vi "Wait for Completion.vi"(8 "error in (no error)":errorcluster, 9 "Timeout":i32, 11 "Coverage Analyzer Process in":refnum<class "Coverage Analyzer Process.lvclass">) -> (0 "error out":errorcluster, 3 "Coverage Analyzer Process out":refnum<class "Coverage Analyzer Process.lvclass">)   [LabVIEW 2020, in "Coverage Analyzer Process.lvclass"]
uses:
  Coverage Analyzer Process.lvclass
  Coverage Analyzer Process.lvclass/Coverage Analyzer Process.ctl
  Coverage Analyzer Result View/Coverage Analyzer View Data.ctl
  Coverage Analyzer Result View/Coverage Analyzer View.vi
  Coverage Analyzer Result View/Coverage Analyzer Result View.lvclass
  Coverage Analyzer/Coverage Analyzer.lvclass
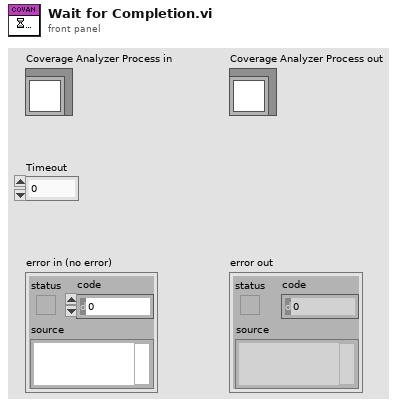
[diagram p1: front panel]
types:
  T1 = typedef "Coverage Analyzer Result View.lvclass/Coverage Analyzer View Data.ctl" = cluster{"Code Coverage":map{path, dbl}}
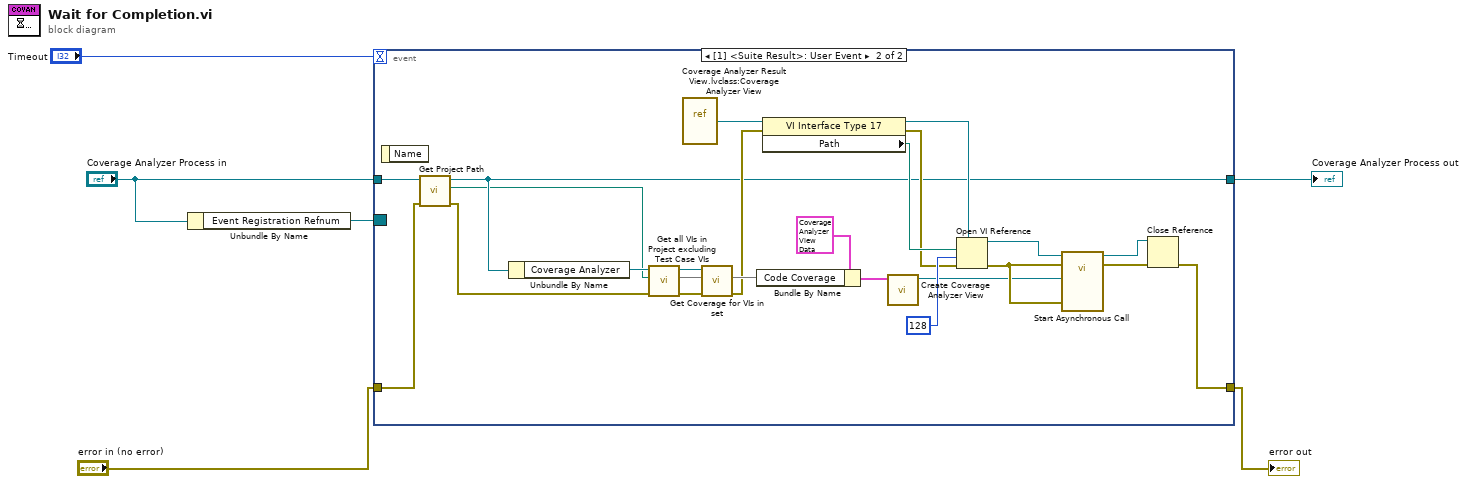
[diagram p0: block diagram]
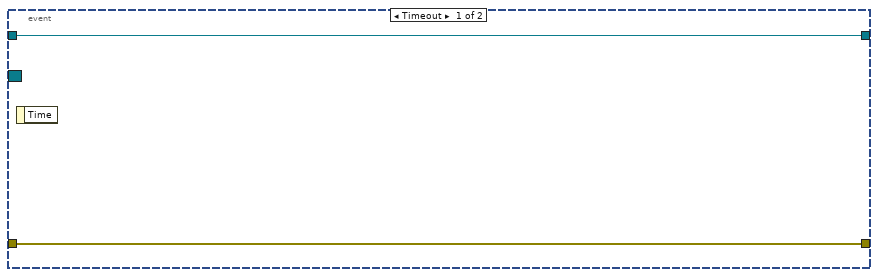
[diagram p2: hidden frame]
diagram:
  n1 = Unbundle By Name("Coverage Analyzer Process in") -> ("Event Registration Refnum"=w5:refnum<event-registration>)
  n2 = event shown="[1] <Suite Result>: User Event" {
    selector: w5 -> [_ _]
    dyn-events: _ -> [_ _]
    timeout: "Timeout" -> [_ _]
    tunnel: "error in (no error)" -> [w8 w13]
    tunnel: [w8 w23] -> w3
    tunnel: "Coverage Analyzer Process in" -> [w7 w15]
    tunnel: [w7 w16] -> w1
    event Timeout {
      n3 = event-data() -> ()  [unwired: 1 in, 1 out]
    }
    event User Event {
      n4 = event-data() -> ()  [unwired: 1 in, 1 out]
      n5 = call "Get Project Path.vi"("error in (no error)"=w13, "Coverage Analyzer Process in"=w15) -> ("error out"=w14:errorcluster, "Path"=w10:path, "Coverage Analyzer Process out"=w16:refnum<class "Coverage Analyzer Process.lvclass">)  [unwired: 7 in]
      n6 = Unbundle By Name(w16) -> ("Coverage Analyzer"=w21:refnum<class "Coverage Analyzer.lvclass">)
      n7 = call "Get all VIs in Project excluding Test Case VIs.vi"("error in (no error)"=w14, "Path"=w10, "Coverage Analyzer in"=w21) -> ("error out"=w18:errorcluster, "VIs"=w9:set{path}, "Coverage Analyzer out"=w20:refnum<class "Coverage Analyzer.lvclass">)  [unwired: 6 in]
      n8 = vi-ref "Coverage Analyzer Result View.lvclass:Coverage Analyzer View.vi"() -> (w25:refnum<vi>)
      n9 = call "Get Coverage for VIs in set.vi"("error in (no error)"=w18, "VIs"=w9, "Coverage Analyzer in"=w20) -> ("error out"=w17:errorcluster, "Code Coverage"=w19:map{path, dbl})  [unwired: 6 in, 1 out]
      n10 = Bundle By Name(cluster=T1 {"Code Coverage"={}} ("Data"), "Code Coverage"=w19) -> (w12:T1)
      n11 = property class="VI Interface Type 17"(reference=w25, error in=w17) -> (reference out=w29:refnum<vi>, error out=w27:errorcluster, "Path"=w28:path)
      n12 = call "Create Coverage Analyzer View.vi"("Coverage Analyzer Result View in"=w12) -> ("Coverage Analyzer Result View out"=w11:refnum<class "Coverage Analyzer Result View.lvclass">)  [unwired: 9 in, 1 out]
      n13 = Open VI Reference(type specifier VI Refnum (for type only)=w29, vi path=w28, options=128, error in (no error)=w27) -> (vi reference=w24:refnum<vi>, error out=w26:errorcluster)  [unwired: 2 in]
      n14 = call-by-ref "Start Asynchronous Call"(reference=w24, error in=w26, 8:"error in (no error)"=w26, "Coverage Analyzer Result View.lvclass"=w11) -> (reference out=w32:refnum<vi>, error out=w31:errorcluster)  [unwired: 9 in, 1 out]
      n15 = Close Reference(reference=w32, error in (no error)=w31) -> (error out=w23:errorcluster)
    }
  }
  "error out" <- w3
  "Coverage Analyzer Process out" <- w1
